vi "公式写入.vi"(7 "公式":cluster{"X^2":dbl, "X":dbl, "b":dbl}, 8 "Error in":errorcluster caption="Error in (no error)") -> (0 "error out":errorcluster)   [LabVIEW 2016, in "CODCr库.lvlib"]
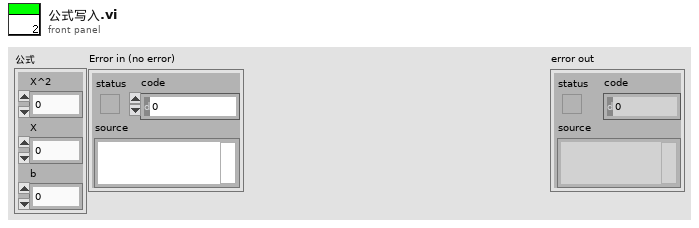
[diagram p1: front panel]
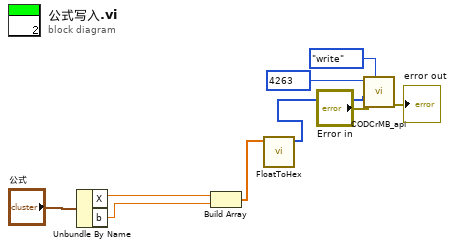
[diagram p0: block diagram]
diagram:
  n1 = Unbundle By Name("公式") -> ("X"=w4:dbl, "b"=w3:dbl)
  n2 = Build Array(w4, w3) -> (w9:dbl[])
  n3 = call "FloatToHex.vi"("浮点数"=w9) -> ("DCBA整形输出"=w6:u16[])  [unwired: 10 in]
  n4 = call "CODCrMB_api.vi"("STEP"=enum16{"open", "read", "write", "close"}."write", "Error in"="Error in", "values"=w6, "starting address"=u16 4263) -> ("error out"=→"error out":errorcluster)  [unwired: 5 in, 2 out]
